vi "Amira Bladder Calibration V0.2 - old.vi"() -> ()   [LabVIEW 2020]
uses:
  <userlib>/KQD LabVIEW User/Serial/Controls/SERIAL PortConfig.ctl
  <userlib>/KQD LabVIEW User/Serial/Controls/SERIAL BaudRate.ctl
  <userlib>/Amira UART/Public/TypeDefs/AUART StepDir.ctl
  <vilib>/Utility/file.llb/Write Delimited Spreadsheet (string).vi
  <userlib>/Amira UART/Amira UART.lvclass
  <userlib>/KQD LabVIEW User/Serial/Serial.lvlib
panel:
  out "Data":dbl[][](graph)
  in  "Iteration":i32
  in  "RunWith":cluster{"Steps":i32, "Rates":i32}={"Steps"=400, "Rates"=40}
  in  "Folder":path=path "C:/Amira Data/Strip"
  in  "StartAt":cluster{"Steps":i32, "Rates":i32}={"Steps"=950, "Rates"=200}
  out "Position":dbl[](graph)
  in  "DAQ":tag="Dev1/port0"
  out "UART":string
  in  "ComPort":refnum<visa-resource-name>
  in  "Config":T1={"BaudRate"=enum."460800", "StopBits"=10, "DataBits"=8, "Parity"=enum."None", "FlowControl"=2, "TimeOut"=1000, "TermChar"=10, "ReadTermEn"=TRUE} {"TermChar" format="%.0x"; "FlowControl" items=["None", "XON/XOFF", "RTS/CTS", "XON/XOFF & RTS/CTS", "DTR/DSR", "XON/XOFF & DTR/DSR"]; "DataBits" min=5 max=8 step=1; "StopBits" items=["1.0"=10, "1.5"=15, "2.0"=20]}
  out "ErrOut":errorcluster
  in  "ErrIn":errorcluster
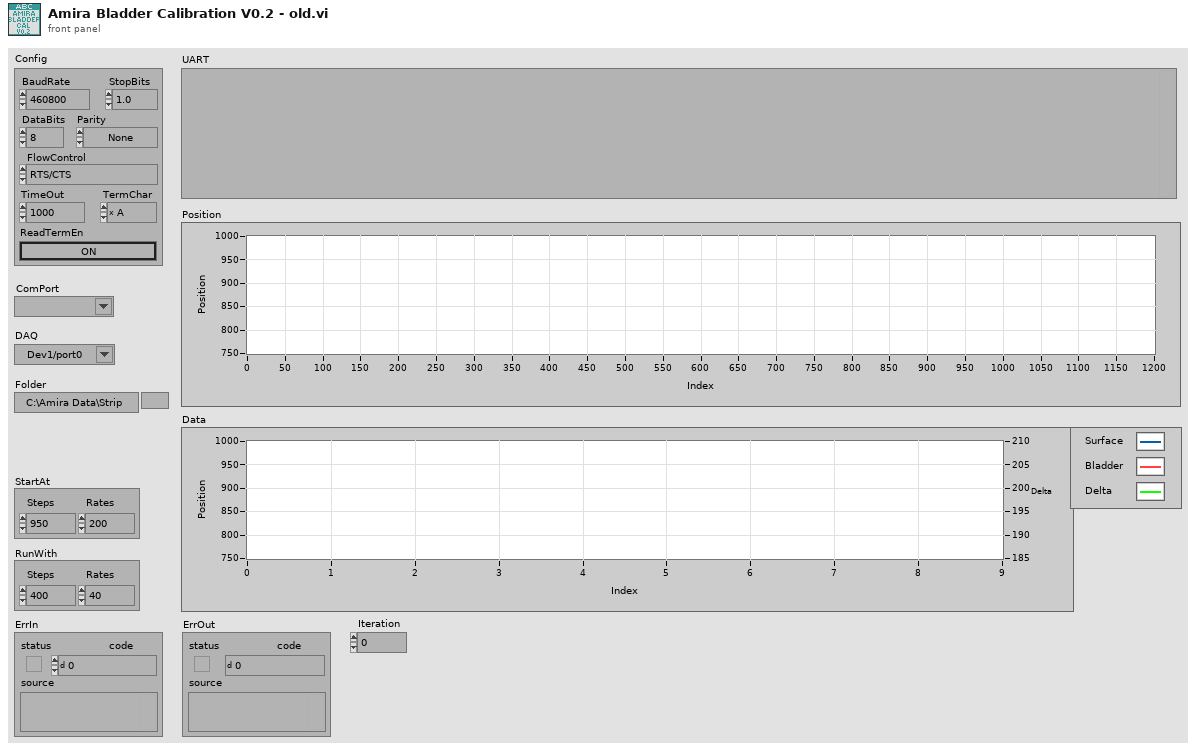
[diagram p1: front panel]
types:
  T1 = typedef "Serial.lvlib/SERIAL PortConfig.ctl" = cluster{"BaudRate":T2, "StopBits":u16, "DataBits":u16, "Parity":enum16{"None", "Odd", "Even", "Mark", "Space"}, "FlowControl":u16, "TimeOut":u32, "TermChar":u8, "ReadTermEn":bool}
  T2 = typedef "SERIAL BaudRate.ctl" = enum16{"2400", "4800", "7200", "9600", "14400", "19200", "28800", "38400", "57600", "115200", "128000", "230400", "460800", "921600"}
  T3 = typedef "Amira UART.lvclass/AUART StepDir.ctl" = enum16{"", "compress", "decompress"}
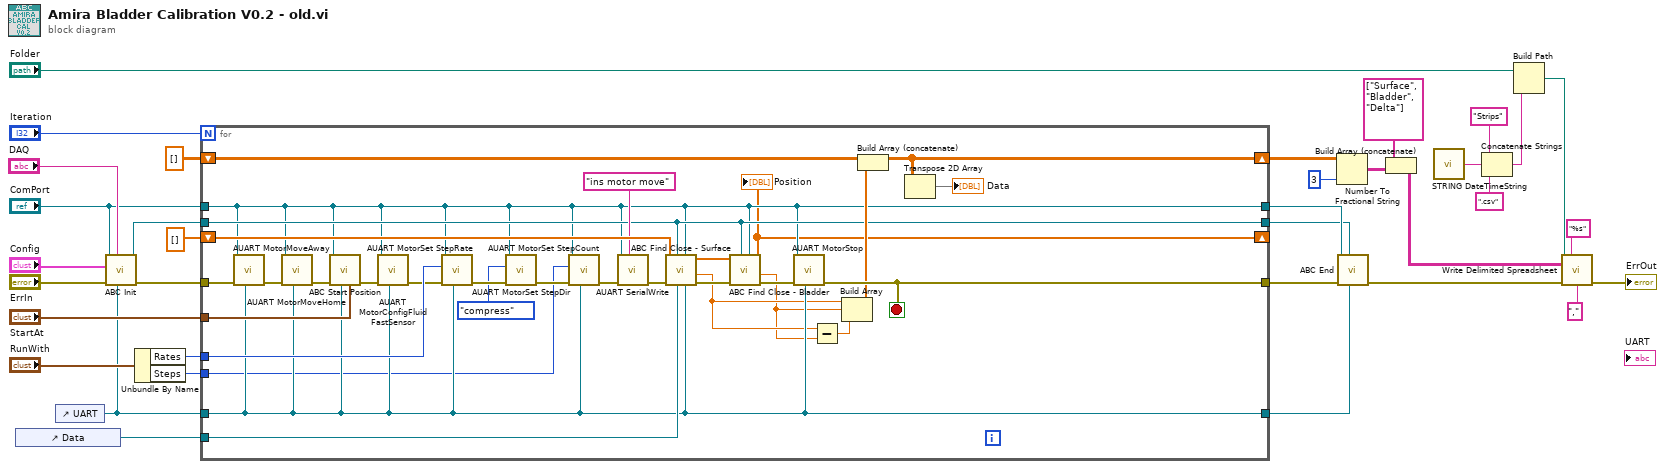
[diagram p0: block diagram]
diagram:
  n1 = control-ref of="Data"() -> (w29:refnum<vi>)
  n2 = control-ref of="UART"() -> (w24:refnum<vi>)
  n3 = call "ABC Init.vi"("UART"=w24, "DAQ"="DAQ", "ErrIn"="ErrIn", "PortConfig"="Config", "ComPort"="ComPort") -> ("ErrOut"=w25:errorcluster, "DaqTask"=w30:refnum<k21>)  [unwired: 5 in]
  n4 = Unbundle By Name("RunWith") -> ("Rates"=w27:i32, "Steps"=w26:i32)
  n5 = for {
    N: "Iteration" -> [_]
    tunnel: "StartAt" -> [w65]
    tunnel: w29 -> [w64]
    tunnel: w27 -> [w63]
    tunnel: w26 -> [w47]
    tunnel: "ComPort" -> [w41]
    tunnel: [w41] -> w21
    tunnel: w30 -> [w42]
    tunnel: [w42] -> w20
    tunnel: w25 -> [w52]
    tunnel: [w61] -> w22
    tunnel: w24 -> [w48]
    tunnel: [w48] -> w18
    shift-right: [w39] -> _
    shift-left: dbl[] [] ("DataOut") -> [w62]
    shift-right: [w59] -> w13
    shift-left: dbl[][] [] -> [w58]
    stop <- w61 stop-if-true
    n6 = call <userlib>:"AUART MotorMoveAway.vi"("UART"=w48, "ErrIn"=w52, "Port"=w41) -> ("ErrOut"=w53:errorcluster)  [unwired: 8 in]
    n7 = call <userlib>:"AUART MotorMoveHome.vi"("UART"=w48, "ErrIn"=w53, "Port"=w41) -> ("ErrOut"=w55:errorcluster)  [unwired: 7 in, 1 out]
    n8 = call "ABC Start Position.vi"("Start"=w65, "UART"=w48, "ErrIn"=w55, "ComPort"=w41) -> ("ErrOut"=w54:errorcluster)  [unwired: 6 in, 1 out]
    n9 = call <userlib>:"AUART MotorConfigFluidFastSensor.vi"("UART"=w48, "ErrIn"=w54, "Port"=w41) -> ("ErrOut"=w56:errorcluster)  [unwired: 8 in]
    n10 = call <userlib>:"AUART MotorSet StepRate.vi"("UART"=w48, "ErrIn"=w56, "step_rate"=w63, "Port"=w41) -> ("ErrOut"=w51:errorcluster)  [unwired: 7 in]
    n11 = call <userlib>:"AUART MotorSet StepDir.vi"("ErrIn"=w51, "step_dir"=AUART_StepDir."compress", "Port"=w41) -> ("ErrOut"=w49:errorcluster)  [unwired: 8 in]
    n12 = call <userlib>:"AUART MotorSet StepCount.vi"("UART"=w48, "ErrIn"=w49, "step_count"=w47, "Port"=w41) -> ("ErrOut"=w46:errorcluster)  [unwired: 7 in]
    n13 = call <userlib>:"AUART SerialWrite.vi"("Cmd"="ins motor move", "ErrIn"=w46, "Port"=w41) -> ("ErrOut"=w44:errorcluster)  [unwired: 7 in, 1 out]
    n14 = call "ABC Find Close - Surface.vi"("UART"=w48, "ComPort"=w41, "Data"=w64, "DaqTask"=w42, "ErrIn"=w44, "DataIn"=w62) -> ("ErrOut"=w43:errorcluster, "SurPos"=w37:dbl, "DataOut"=w40:dbl[])  [unwired: 3 in]
    n15 = call "ABC Find Close - Bladder.vi"("ComPort"=w41, "DaqTask"=w42, "ErrIn"=w43, "DataIn"=w40) -> ("ErrOut"=w38:errorcluster, "BlaPos"=w36:dbl, "DataOut"=w39:dbl[])  [unwired: 5 in]
    "Position" <- w39
    n16 = call <userlib>:"AUART MotorStop.vi"("UART"=w48, "ErrIn"=w38, "Port"=w41) -> ("ErrOut"=w61:errorcluster)  [unwired: 8 in]
    n17 = Subtract(x=w37, y=w36) -> (x-y=w35:dbl)
    n18 = Build Array(w37, w36, w35) -> (w60:dbl[])
    n19 = Build Array (concatenate)(w58, w60) -> (w59:dbl[][])
    n20 = Transpose 2D Array(2D array=w59) -> (transposed array=→"Data":dbl[][])
  }
  n21 = Number To Fractional String(number=w13, precision (6)=i16 3) -> (F-format string=w11:string[][])  [unwired: 2 in]
  n22 = call "ABC End.vi"("UART"=w18, "DaqTask"=w20, "ErrIn"=w22, "ComPort"=w21) -> ("ErrOut"=w15:errorcluster)  [unwired: 7 in]
  n23 = Build Array (concatenate)(string[] ["Surface", "Bladder", "Delta"], w11) -> (w9:string[][])
  n24 = call <userlib>:"STRING DateTimeString.vi"() -> ("DateTimeStr"=w5:string)  [unwired: 2 in]
  n25 = Concatenate Strings("Strips" ("string"), w5, ".csv" ("string")) -> (w3:string)
  n26 = Build Path(base path="Folder", name or relative path=w3) -> (appended path=w2:path)
  n27 = call-poly <vilib>:"Write Delimited Spreadsheet.vi"("file path (dialog if empty)"=w2, "format (%s)"="%s", "2D data"=w9, "error in (no error)"=w15, "delimiter (\\t)"="," ("delimiter (\\t)")) -> ("error out"=→"ErrOut":errorcluster)  [unwired: 9 in, 1 out]
